vi "Periodic Tasks.vi"(8 "error in (no error)":errorcluster) -> ()   [LabVIEW 2014]
doc: "This VI runs in parallel to other tasks. It can contain as many user-defined periodic loops as you need. These can carry out PID or other sorts of timed response."
panel:
  out "Waveform Z":dbl(graph)
  out "Waveform Y":dbl(graph)
  out "Waveform X":dbl(graph)
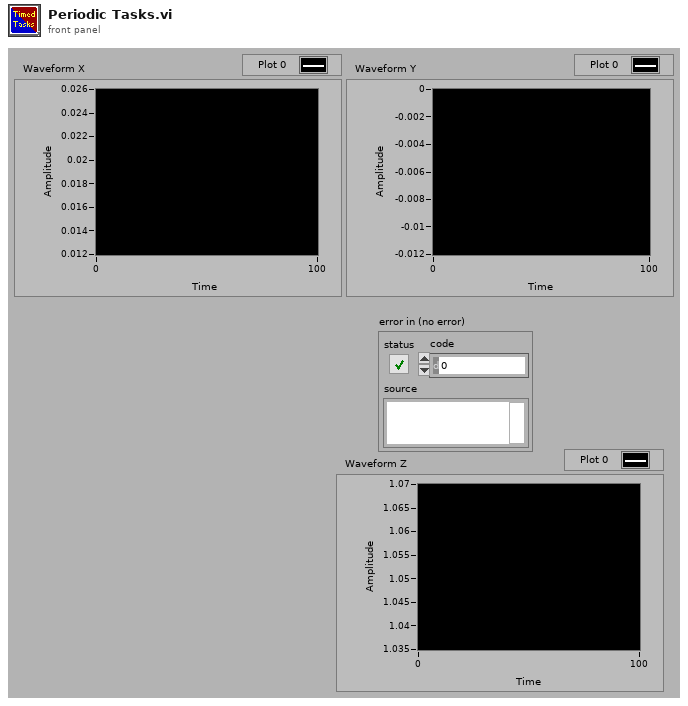
[diagram p1: front panel]
types:
  T1 = typedef "WPI_CameraDevRef.ctl" = cluster{"Camera Address":string, "CameraStatus":errorcluster}
  T2 = cluster{"X-Axis":dbl, "Y-Axis":dbl, "Z-Axis":dbl}
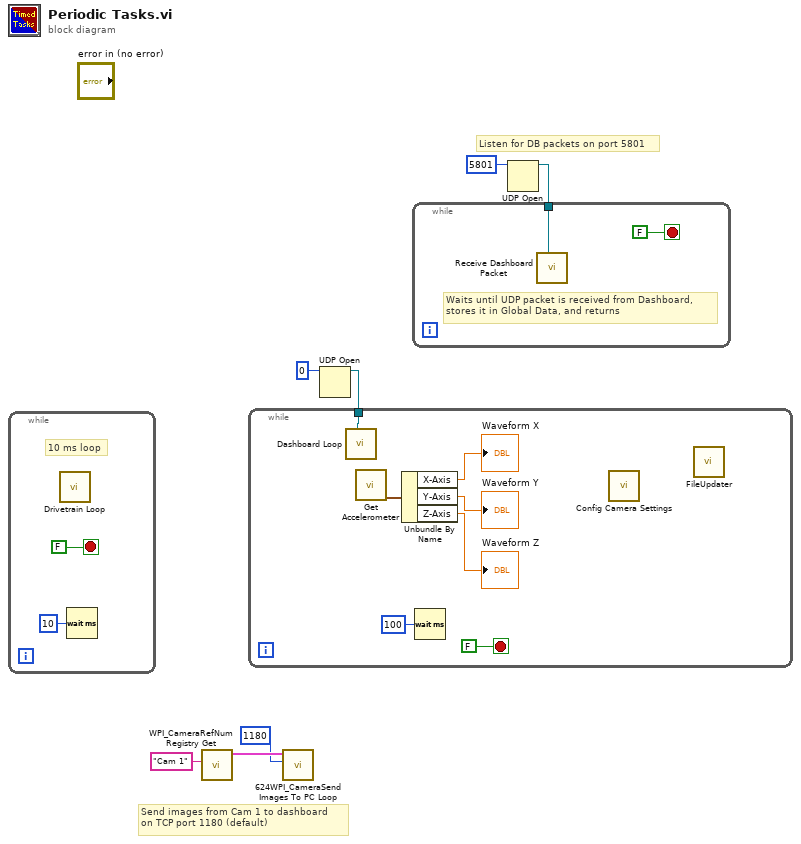
[diagram p0: block diagram]
diagram:
  # "Send images from Cam 1 to dashboard\non TCP port 1180 (default)"
  # "Listen for DB packets on port 5801"
  n1 = while {
    stop <- FALSE stop-if-true
    # "10 ms loop"
    n2 = call "Drivetrain Loop.vi"() -> ()  [unwired: 12 in]
    n3 = Wait (ms)(milliseconds to wait=u32 10) -> ()  [unwired: 1 out]
  }
  n4 = call <vilib>:"WPI_CameraRefNum Registry Get.vi"("refnum name"="Cam 1") -> ("CameraDevRef"=w2:T1)  [unwired: 9 in, 1 out]
  n5 = call "624WPI_CameraSend Images To PC Loop.vi"("port"=u16 1180, "CameraDevRef"=w2) -> ()  [unwired: 10 in]
  n6 = UDP Open(11:u16 0 ("port")) -> (port=w5:refnum<k16>)  [unwired: 4 in, 2 out]
  n7 = while {
    tunnel: w5 -> [w14]
    stop <- FALSE stop-if-true
    n8 = call "Dashboard Loop.vi"("connection ID"=w14) -> ()  [unwired: 11 in]
    n9 = call "Get Accelerometer.vi"() -> ("Accelerations"=w10:T2)  [unwired: 11 in]
    n10 = Unbundle By Name(w10) -> ("X-Axis"=→"Waveform X":dbl, "Y-Axis"=→"Waveform Y":dbl, "Z-Axis"=→"Waveform Z":dbl)
    n11 = Wait (ms)(milliseconds to wait=u32 100) -> ()  [unwired: 1 out]
    n12 = call "Config Camera Settings.vi"() -> ()  [unwired: 12 in]
    n13 = call "FileUpdater.vi"() -> ()  [unwired: 12 in]
  }
  n14 = UDP Open(11:u16 5801 ("port")) -> (port=w7:refnum<k16>)  [unwired: 4 in, 2 out]
  n15 = while {
    tunnel: w7 -> [w17]
    stop <- FALSE stop-if-true
    # "Waits until UDP packet is received from Dashboard,\nstores it in Global Data, and returns"
    n16 = call "Receive Dashboard Packet.vi"("connection ID"=w17) -> ()  [unwired: 11 in]
  }
